vi "CMD_DIALOG.vi"(7 "Console Log in":refnum<class "Console Log.lvclass">, 8 "error in (no error)":errorcluster, 10 "Arguments":string[](array[string]), 11 "gScript Interpreter in":refnum<class "gScript Interpreter.lvclass">) -> (0 "error out":errorcluster, 3 "gScript Interpreter out":refnum<class "gScript Interpreter.lvclass">, 5 "Console Log out":refnum<class "Console Log.lvclass">)   [LabVIEW 2022 SP3, in "gScript Interpreter.lvclass"]
uses:
  gScript Interpreter.lvclass
  Application Utilities/Console Log/Console Log.lvclass
  <vilib>/Utility/miscctls.llb/LVRectTypeDef.ctl
  <vilib>/Utility/miscctls.llb/LVPointTypeDef.ctl
  <vilib>/Utility/config.llb/Read Key (U32).vi
  <vilib>/Utility/config.llb/Read Key (String).vi
  <vilib>/Utility/config.llb/Read Key (I32).vi
  <vilib>/Utility/config.llb/Read Key (Boolean).vi
  <vilib>/Utility/config.llb/Read Key (Double).vi
  <vilib>/Utility/config.llb/NI_LVConfig.lvlib
panel:
  in  "float_input_10":dbl caption="Numeric"
  in  "float_input_9":dbl caption="Numeric"
  in  "float_input_8":dbl caption="Numeric"
  in  "float_input_7":dbl caption="Numeric"
  in  "float_input_6":dbl caption="Numeric"
  in  "float_input_5":dbl caption="Numeric"
  in  "float_input_4":dbl caption="Numeric"
  in  "float_input_3":dbl caption="Numeric"
  in  "float_input_2":dbl caption="Hello World"
  in  "float_input_1":dbl caption="Hello World"
  in  "int_input_10":i32 caption="int_control_1"
  in  "int_input_9":i32 caption="int_control_1"
  in  "int_input_8":i32 caption="int_control_1"
  in  "int_input_7":i32 caption="int_control_1"
  in  "int_input_6":i32 caption="int_control_1"
  in  "int_input_5":i32 caption="int_control_1"
  in  "int_input_4":i32 caption="int_control_1"
  in  "int_input_3":i32 caption="int_control_1"
  in  "int_input_2":i32 caption="int_control_1"
  in  "int_input_1":i32 caption="int_control_1"
  in  "bool_input_10":bool
  in  "bool_input_9":bool
  in  "bool_input_8":bool
  in  "bool_input_7":bool
  in  "bool_input_6":bool
  in  "bool_input_5":bool
  in  "bool_input_4":bool
  in  "bool_input_3":bool
  in  "bool_input_2":bool caption="Hello World 2"
  in  "bool_input_1":bool caption="Hello World"
  in  "continue":bool
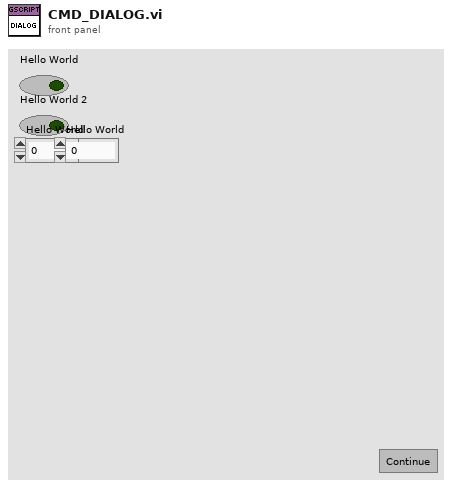
[diagram p1: front panel]
types:
  T1 = typedef "LVRectTypeDef.ctl" = cluster{"Left":i16, "Top":i16, "Right":i16, "Bottom":i16}
  T2 = typedef "LVPointTypeDef.ctl" = cluster{"Horizontal":i16, "Vertical":i16}
  T3 = typedef "NI_LVConfig.lvlib/Config Data RefNum.ctl" = refnum<k1>
  T4 = typedef "Memory Cell.ctl" = cluster{"type":T5, "x":dbl, "y":dbl, "z":dbl, "w":dbl}
  T5 = typedef "Memory Cell Type Enum.ctl" = enum16{"integer", "float", "vector", "rotation"}
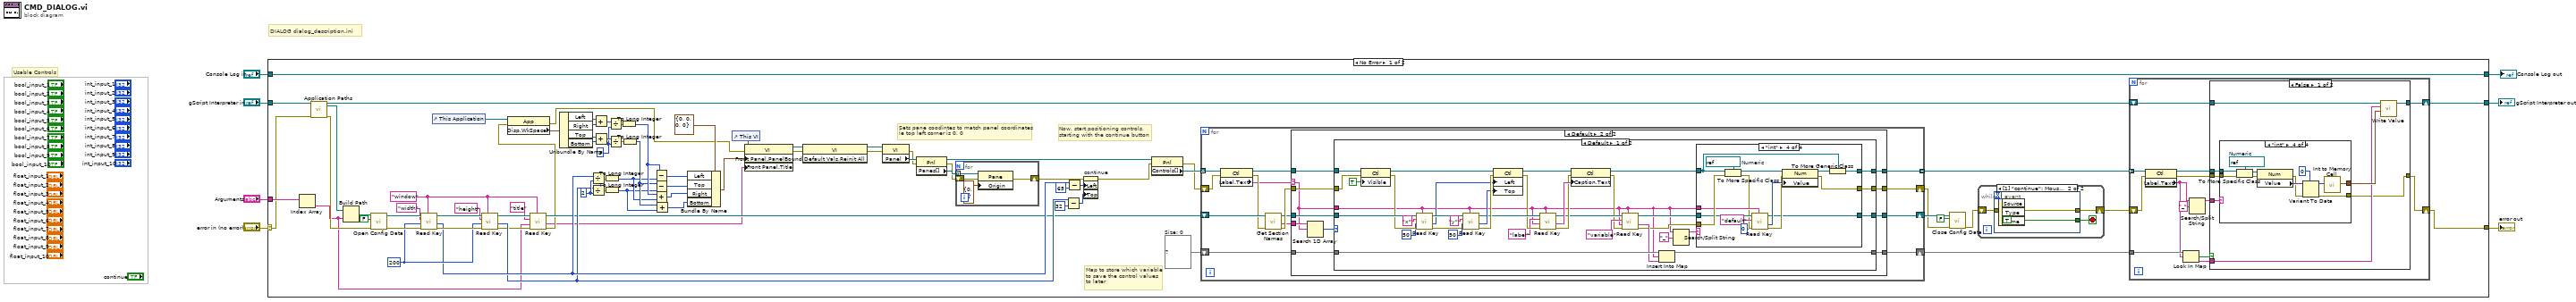
[diagram p0: block diagram]
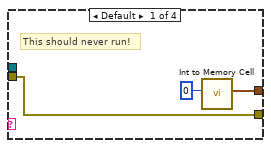
[diagram p2: hidden frame]
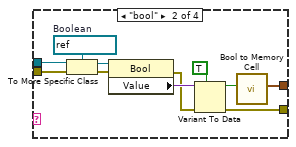
[diagram p3: hidden frame]
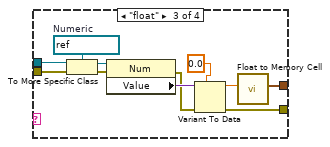
[diagram p4: hidden frame]
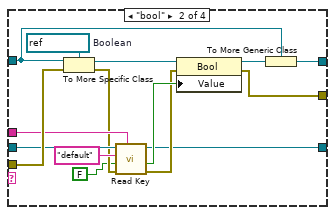
[diagram p8: hidden frame]
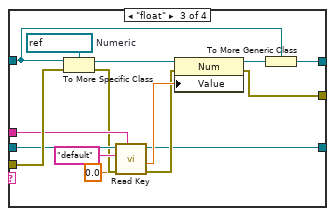
[diagram p9: hidden frame]
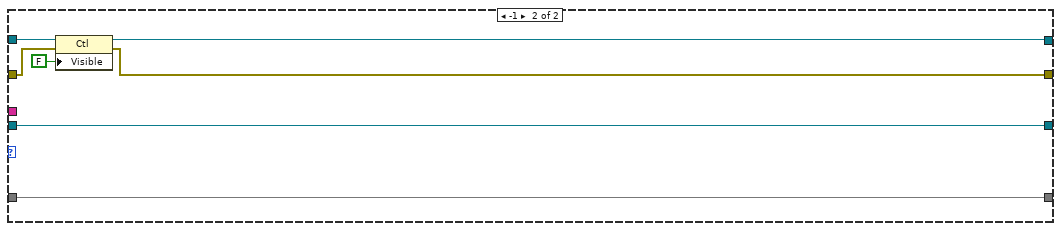
[diagram p10: hidden frame]
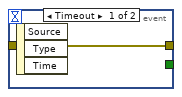
[diagram p11: hidden frame]
diagram:
  # "Usable Controls"
  # "DIALOG dialog_description.ini"
  n1 = case shown="No Error" "error in (no error)" {
    selector: "error in (no error)" -> [w84 w278]
    tunnel: [w9 w278] -> w6
    tunnel: [w10 w277] -> w4
    tunnel: "gScript Interpreter in" -> [w85 w277]
    tunnel: "Arguments" -> [w86 _]
    tunnel: "Console Log in" -> [w8 w276]
    tunnel: [w8 w276] -> w1
    frame No Error {
      w16 = map{string, string} {}  # Size: 0
      w56 = 2
      w61 = 2
      w72 = u32 200 ("default value")
      w22 = "window" ("section")
      # "Map to store which variable\nto save the control values\nto later"
      # "Now, start positioning controls, \nstarting with the continue button"
      # "Sets pane coodintes to match panel coordinates\nie top left corner is 0, 0"
      n2 = Index Array(array=w86) -> (element=w18:string)  [unwired: 1 in]
      n3 = call "Application Paths.vi"("gScript Interpreter in"=w85, "error in (no error)"=w84) -> ("gScript Interpreter out"=w11:refnum<class "gScript Interpreter.lvclass">, "Project Path"=w83:path, "error out"=w81:errorcluster)  [unwired: 12 in, 3 out]
      n4 = Build Path(base path=w83, name or relative path=w18) -> (appended path=w82:path)
      n5 = call <vilib>:"Open Config Data.vi"("error in (no error)"=w81, "create file if necessary (T)"=FALSE, "configuration file path"=w82) -> ("error out"=w77:errorcluster, "refnum"=w79:T3)  [unwired: 6 in, 1 out]
      n6 = call-poly <vilib>:"Read Key.vi"("section"=w22, "error in (no error)"=w77, "default value"=w72, "key"="width", "refnum"=w79) -> ("error out"=w75:errorcluster, "value"=w38:u32, "refnum out"=w76:T3)  [unwired: 3 in, 1 out]
      n7 = control-ref of="This Application"() -> (w69:refnum<vi>)
      n8 = call-poly <vilib>:"Read Key.vi"("section"=w22, "error in (no error)"=w75, "default value"=w72, "key"="height", "refnum"=w76) -> ("error out"=w20:errorcluster, "value"=w37:u32, "refnum out"=w23:T3)  [unwired: 3 in, 1 out]
      n9 = call-poly <vilib>:"Read Key.vi"("section"=w22, "error in (no error)"=w20, "default value"=w18, "key"="title", "refnum"=w23) -> ("error out"=w19:errorcluster, "value"=w17:string, "refnum out"=w24:T3)  [unwired: 3 in, 1 out]
      n10 = property class="App"(reference=w69, error in=w19) -> (error out=w48:errorcluster, "Disp.WkSpace"=w68:T1)  [unwired: 1 out]
      n11 = Unbundle By Name(w68) -> ("Left"=w67:i16, "Right"=w66:i16, "Top"=w64:i16, "Bottom"=w63:i16)
      n12 = Divide(x=w38, y=w56) -> (x/y=w58:dbl)
      n13 = Divide(x=w37, y=w56) -> (x/y=w57:dbl)
      n14 = Add(x=w67, y=w66) -> (x+y=w65:i16)
      n15 = Add(x=w64, y=w63) -> (x+y=w62:i16)
      n16 = To Long Integer(number=w58) -> (32bit integer=w47:i32)
      n17 = To Long Integer(number=w57) -> (32bit integer=w46:i32)
      n18 = Divide(x=w65, y=w61) -> (x/y=w60:dbl)
      n19 = Divide(x=w62, y=w61) -> (x/y=w59:dbl)
      n20 = To Long Integer(number=w60) -> (32bit integer=w52:i32)
      n21 = To Long Integer(number=w59) -> (32bit integer=w50:i32)
      n22 = Subtract(x=w52, y=w47) -> (x-y=w55:i32)
      n23 = Subtract(x=w50, y=w46) -> (x-y=w54:i32)
      n24 = Add(x=w52, y=w47) -> (x+y=w53:i32)
      n25 = Add(x=w50, y=w46) -> (x+y=w51:i32)
      n26 = Bundle By Name(cluster=T1 {"Left"=0, "Top"=0, "Right"=0, "Bottom"=0} ("Front Panel Window:Window Bounds"), "Left"=w55, "Top"=w54, "Right"=w53, "Bottom"=w51) -> (w45:T1)
      n27 = control-ref of="This VI"() -> (w73:refnum<vi>)
      n28 = property class="VI"(reference=w73, error in=w48, "Front Panel.PanelBounds"=w45, "Front Panel.Title"=w17) -> (reference out=w33:refnum<vi>, error out=w32:errorcluster)
      n29 = invoke class="VI" method="Default Vals.Reinit All"(reference=w33, error in=w32) -> (reference out=w31:refnum<vi>, error out=w30:errorcluster)  [unwired: 1 in, 1 out]
      n30 = property class="VI"(reference=w31, error in=w30) -> (error out=w39:errorcluster, "Panel"=w40:refnum<vi>)  [unwired: 1 out]
      n31 = property class="Pnl"(reference=w40, error in=w39) -> (reference out=w29:refnum<vi>, error out=w35:errorcluster, "Panes[]"=w36:refnum<vi>[])
      n32 = for {
        tunnel: w36 -> [w269] mode=indexing
        shift-right: [w266] -> w34
        shift-left: w35 -> [w267]
        n33 = property class="Pane"(reference=w269, error in=w267, "Origin"=T2 {"Horizontal"=0, "Vertical"=0}) -> (error out=w266:errorcluster)  [unwired: 1 out]
      }
      n34 = Subtract(x=w37, y=u32 32) -> (x-y=w41:u32)
      n35 = Subtract(x=w38, y=u32 65) -> (x-y=w44:u32)
      n36 = property on="continue" class="Bool (strict)"(error in=w34, "Left"=w44, "Top"=w41) -> (error out=w28:errorcluster)  [unwired: 1 in, 1 out]
      n37 = property class="Pnl"(reference=w29, error in=w28) -> (error out=w25:errorcluster, "Controls[]"=w26:refnum<vi>[])  [unwired: 1 out]
      n38 = for {
        shift-right: [w155] -> w27
        shift-left: w24 -> [w154]
        tunnel: w26 -> [w159] mode=indexing
        shift-right: [w156] -> w15
        shift-left: w25 -> [w158]
        shift-right: [w147] -> w13
        shift-left: w16 -> [w148]
        tunnel: [w146] -> w14 mode=indexing
        n39 = property class="Ctl"(reference=w159, error in=w158) -> (reference out=w157:refnum<vi>, error out=w153:errorcluster, "Label.Text"=w149:string)
        n40 = call <vilib>:"Get Section Names.vi"("error in (no error)"=w153, "refnum"=w154) -> ("error out"=w152:errorcluster, "section names"=w150:string[], "refnum out"=w151:T3)  [unwired: 7 in]
        n41 = case shown="Default" w149 {
          selector: w149 -> [_ w167]
          tunnel: w157 -> [w160 w172]
          tunnel: w152 -> [w163 w170]
          tunnel: [w163 w168] -> w156
          tunnel: w151 -> [w162 w171]
          tunnel: [w162 w169] -> w155
          tunnel: w150 -> [_ w174]
          tunnel: w148 -> [w161 w166]
          tunnel: [w161 w165] -> w147
          tunnel: [w160 w164] -> w146
          frame "continue" {
          }
          frame Default {
            n42 = Search 1D Array(1D array=w174, element=w167) -> (index of element=w173:i32)  [unwired: 1 in]
            n43 = case shown="Default" w173 {
              tunnel: w172 -> [w209 w265]
              tunnel: w171 -> [w207 w262]
              tunnel: w170 -> [w208 w263]
              tunnel: [w177 w262] -> w169
              tunnel: [w176 w261] -> w168
              tunnel: w167 -> [w178 _]
              tunnel: w166 -> [w186 w260]
              tunnel: [w184 w260] -> w165
              tunnel: [w175 w259] -> w164
              frame Default {
                n44 = property class="Ctl"(reference=w209, error in=w208, "Visible"=TRUE) -> (reference out=w199:refnum<vi>, error out=w206:errorcluster)
                n45 = call-poly <vilib>:"Read Key.vi"("section"=w178, "error in (no error)"=w206, "default value"=50, "key"="x", "refnum"=w207) -> ("error out"=w200:errorcluster, "value"=w197:i32, "refnum out"=w201:T3)  [unwired: 3 in, 1 out]
                n46 = call-poly <vilib>:"Read Key.vi"("section"=w178, "error in (no error)"=w200, "default value"=50, "key"="y", "refnum"=w201) -> ("error out"=w198:errorcluster, "value"=w196:i32, "refnum out"=w195:T3)  [unwired: 3 in, 1 out]
                n47 = property class="Ctl"(reference=w199, error in=w198, "Left"=w197, "Top"=w196) -> (reference out=w192:refnum<vi>, error out=w194:errorcluster)
                n48 = call-poly <vilib>:"Read Key.vi"("section"=w178, "error in (no error)"=w194, "default value"=w178, "key"="label", "refnum"=w195) -> ("error out"=w190:errorcluster, "value"=w191:string, "refnum out"=w188:T3)  [unwired: 3 in, 1 out]
                n49 = property class="Ctl"(reference=w192, error in=w190, "Caption.Text"=w191) -> (reference out=w179:refnum<vi>, error out=w187:errorcluster)
                n50 = call-poly <vilib>:"Read Key.vi"("section"=w178, "error in (no error)"=w187, "default value"=w178, "key"="variable", "refnum"=w188) -> ("error out"=w180:errorcluster, "value"=w185:string, "refnum out"=w181:T3)  [unwired: 3 in, 1 out]
                n51 = Insert Into Map(map in=w186, key=w178, value=w185) -> (map out=w184:map{string, string})  [unwired: 2 out]
                n52 = Search/Split String(string=w178, search string/char (-)="_") -> (substring before match=w182:string)  [unwired: 1 in, 2 out]
                n53 = case shown="\"int\"" w182 {
                  tunnel: w181 -> [w212 w226 w241 w256]
                  tunnel: w180 -> [w211 w227 w242 w257]
                  tunnel: w179 -> [w213 w216 w232 w247]
                  tunnel: w178 -> [_ w225 w240 w255]
                  tunnel: [w213 w215 w231 w246] -> w175
                  tunnel: [w212 w218 w234 w249] -> w177
                  tunnel: [w211 w214 w230 w245] -> w176
                  frame Default {
                  }
                  frame "bool" {
                    w228 = refnum<vi> refnum  # Boolean
                    n54 = To More Specific Class(target class=w228, reference=w216, error in=w227) -> (specific class reference=w221:refnum<vi>, error out=w223:errorcluster)
                    n55 = call-poly <vilib>:"Read Key.vi"("section"=w225, "error in (no error)"=w223, "default value"=FALSE, "key"="default", "refnum"=w226) -> ("error out"=w219:errorcluster, "value"=w220:bool, "refnum out"=w218:T3)  [unwired: 3 in, 1 out]
                    n56 = property class="Bool"(reference=w221, error in=w219, "Value"=w220) -> (reference out=w217:refnum<vi>, error out=w214:errorcluster)
                    n57 = To More Generic Class(target class=w216, reference=w217) -> (generic class reference=w215:refnum<vi>)
                  }
                  frame "float" {
                    w243 = refnum<vi> refnum  # Numeric
                    n58 = To More Specific Class(target class=w243, reference=w232, error in=w242) -> (specific class reference=w237:refnum<vi>, error out=w238:errorcluster)
                    n59 = call-poly <vilib>:"Read Key.vi"("section"=w240, "error in (no error)"=w238, "default value"=0.0, "key"="default", "refnum"=w241) -> ("error out"=w235:errorcluster, "value"=w236:dbl, "refnum out"=w234:T3)  [unwired: 3 in, 1 out]
                    n60 = property class="Num"(reference=w237, error in=w235, "Value"=w236) -> (reference out=w233:refnum<vi>, error out=w230:errorcluster)
                    n61 = To More Generic Class(target class=w232, reference=w233) -> (generic class reference=w231:refnum<vi>)
                  }
                  frame "int" {
                    w258 = refnum<vi> refnum  # Numeric
                    n62 = To More Specific Class(target class=w258, reference=w247, error in=w257) -> (specific class reference=w252:refnum<vi>, error out=w253:errorcluster)
                    n63 = call-poly <vilib>:"Read Key.vi"("section"=w255, "error in (no error)"=w253, "default value"=0, "key"="default", "refnum"=w256) -> ("error out"=w250:errorcluster, "value"=w251:i32, "refnum out"=w249:T3)  [unwired: 3 in, 1 out]
                    n64 = property class="Num"(reference=w252, error in=w250, "Value"=w251) -> (reference out=w248:refnum<vi>, error out=w245:errorcluster)
                    n65 = To More Generic Class(target class=w247, reference=w248) -> (generic class reference=w246:refnum<vi>)
                  }
                }
              }
              frame -1 {
                n66 = property class="Ctl"(reference=w265, error in=w263, "Visible"=FALSE) -> (reference out=w259:refnum<vi>, error out=w261:errorcluster)
              }
            }
          }
        }
      }
      n67 = call <vilib>:"Close Config Data.vi"("error in (no error)"=w15, "write file if changed (T)"=FALSE, "refnum"=w27) -> ("error out"=w70:errorcluster)  [unwired: 7 in, 1 out]
      n68 = while {
        shift-right: [w270] -> w12
        shift-left: w70 -> [w271]
        stop <- w272 stop-if-true
        n69 = event shown="[1] \"continue\": Mouse Up;  Panel Close" {
          selector: _ -> [_ _]
          dyn-events: _ -> [_ _]
          timeout: _ -> [_ _]
          tunnel: [_ TRUE] -> w272
          tunnel: w271 -> [w273 w274]
          tunnel: [w273 w274] -> w270
          event Timeout {
            n70 = event-data() -> ()  [unwired: 1 in, 3 out]
          }
          event "continue": Mouse Up; Panel Close {
            n71 = event-data() -> ()  [unwired: 1 in, 3 out]
          }
        }
      }
      n72 = for {
        tunnel: w14 -> [w98] mode=indexing
        tunnel: w13 -> [w99]
        shift-right: [w92] -> w9
        shift-left: w12 -> [w97]
        shift-right: [w94] -> w10
        shift-left: w11 -> [w95]
        n73 = property class="Ctl"(reference=w98, error in=w97) -> (reference out=w91:refnum<vi>, error out=w93:errorcluster, "Label.Text"=w89:string)
        n74 = Look In Map(map=w99, key=w89) -> (key not found?=w96:bool, value=w87:string)  [unwired: 1 in]
        n75 = Search/Split String(string=w89, search string/char (-)="_") -> (substring before match=w88:string)  [unwired: 1 in, 2 out]
        n76 = case shown="False" w96 {
          tunnel: w95 -> [w104 w145]
          tunnel: [w103 w145] -> w94
          tunnel: w93 -> [w105 w144]
          tunnel: [w100 w144] -> w92
          tunnel: w91 -> [w106 _]
          tunnel: w88 -> [w107 _]
          tunnel: w87 -> [w101 _]
          frame False {
            n77 = case shown="\"int\"" w107 {
              tunnel: w106 -> [_ w121 w132 w143]
              tunnel: w105 -> [w108 w120 w131 w142]
              tunnel: [w108 w113 w125 w136] -> w100
              tunnel: [w110 w111 w122 w133] -> w102
              frame Default {
                # "This should never run!"
                n78 = call "Int to Memory Cell.vi"("Numeric"=0) -> ("Memory Cell"=w110:T4)  [unwired: 10 in]
              }
              frame "bool" {
                w119 = refnum<vi> refnum  # Boolean
                n79 = To More Specific Class(target class=w119, reference=w121, error in=w120) -> (specific class reference=w118:refnum<vi>, error out=w117:errorcluster)
                n80 = property class="Bool"(reference=w118, error in=w117) -> (error out=w115:errorcluster, "Value"=w116:variant)  [unwired: 1 out]
                n81 = Variant To Data(error in=w115, type=TRUE, Variant=w116) -> (data=w112:bool, error out=w113:errorcluster)
                n82 = call "Bool to Memory Cell.vi"("Boolean in"=w112) -> ("Memory Cell"=w111:T4)  [unwired: 10 in]
              }
              frame "float" {
                w130 = refnum<vi> refnum  # Numeric
                n83 = To More Specific Class(target class=w130, reference=w132, error in=w131) -> (specific class reference=w129:refnum<vi>, error out=w128:errorcluster)
                n84 = property class="Num"(reference=w129, error in=w128) -> (error out=w126:errorcluster, "Value"=w127:variant)  [unwired: 1 out]
                n85 = Variant To Data(error in=w126, type=0.0, Variant=w127) -> (data=w123:dbl, error out=w125:errorcluster)
                n86 = call "Float to Memory Cell.vi"("Float in"=w123) -> ("Memory Cell"=w122:T4)  [unwired: 10 in]
              }
              frame "int" {
                w141 = refnum<vi> refnum  # Numeric
                n87 = To More Specific Class(target class=w141, reference=w143, error in=w142) -> (specific class reference=w140:refnum<vi>, error out=w139:errorcluster)
                n88 = property class="Num"(reference=w140, error in=w139) -> (error out=w137:errorcluster, "Value"=w138:variant)  [unwired: 1 out]
                n89 = Variant To Data(error in=w137, type=0, Variant=w138) -> (data=w134:i32, error out=w136:errorcluster)
                n90 = call "Int to Memory Cell.vi"("Numeric"=w134) -> ("Memory Cell"=w133:T4)  [unwired: 10 in]
              }
            }
            n91 = call-dynamic "Write Value.vi"("Value"=w102, "Address"=w101, "gScript Interpreter in"=w104) -> ("gScript Interpreter out"=w103:refnum<class "gScript Interpreter.lvclass">)  [unwired: 7 in, 1 out]
          }
          frame True {
            # "Not found in dictionary, meaning control is not used so skip it!"
          }
        }
      }
    }
    frame Error {
    }
  }
  "error out" <- w6
  "gScript Interpreter out" <- w4
  "Console Log out" <- w1
